vi "Server.vi"() -> ()   [LabVIEW 2023]
uses:
  <vilib>/OPCUA/controls/Data Type.ctl
  <vilib>/OPCUA/controls/NodeId.ctl
  <vilib>/OPCUA/server/Read Variant.vi
  <vilib>/OPCUA/NI OPC UA Server.lvlib
panel:
  out "Temperature on server":variant
  out "Location on server":variant
  in  "Stop Button":bool
  out "Item Node Ids":string
  out "Server Endpoint URL":string
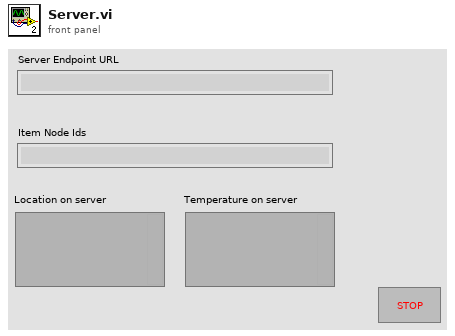
[diagram p1: front panel]
types:
  T1 = typedef "NodeId.ctl" = string
  T2 = typedef "Data Type.ctl" = u16
  T3 = cluster{"name":string, "data type":T2, "access level":u16, "description":string}
  T4 = typedef "OPC UA Server Refnum.ctl" = refnum<k21>
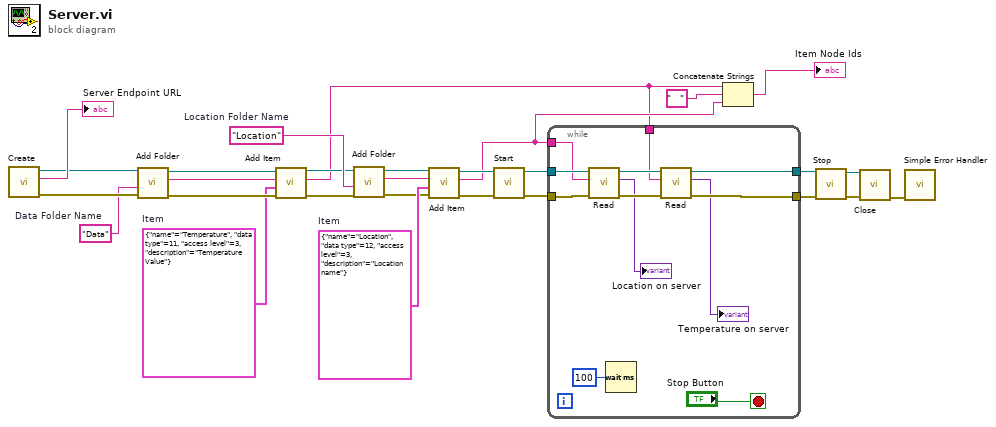
[diagram p0: block diagram]
diagram:
  w8 = "Location"  # Location Folder Name
  w13 = T3 {"name"="Location", "data type"=12, "access level"=3, "description"="Location name"}  # Item
  w16 = T3 {"name"="Temperature", "data type"=11, "access level"=3, "description"="Temperature Value"}  # Item
  w18 = "Data"  # Data Folder Name
  n1 = call <vilib>:"Create.vi"() -> ("error out"=w27:errorcluster, "server endpoint URL"=→"Server Endpoint URL":string, "OPC UA server refnum out"=w21:T4)  [unwired: 9 in]
  n2 = call <vilib>:"Add Folder.vi"("error in (no error)"=w27, "folder name"=w18, "OPC UA server refnum in"=w21) -> ("error out"=w22:errorcluster, "folder node ID"=w17:T1, "OPC UA server refnum out"=w20:T4)  [unwired: 5 in]
  n3 = call <vilib>:"Add Item.vi"("error in (no error)"=w22, "item"=w16, "parent folder node ID"=w17, "OPC UA server refnum in"=w20) -> ("error out"=w10:errorcluster, "item node ID"=w1:T1, "OPC UA server refnum out"=w7:T4)  [unwired: 3 in, 1 out]
  n4 = call <vilib>:"Add Folder.vi"("error in (no error)"=w10, "folder name"=w8, "OPC UA server refnum in"=w7) -> ("error out"=w9:errorcluster, "folder node ID"=w5:T1, "OPC UA server refnum out"=w6:T4)  [unwired: 5 in]
  n5 = call <vilib>:"Add Item.vi"("error in (no error)"=w9, "item"=w13, "parent folder node ID"=w5, "OPC UA server refnum in"=w6) -> ("error out"=w11:errorcluster, "item node ID"=w2:T1, "OPC UA server refnum out"=w12:T4)  [unwired: 3 in, 1 out]
  n6 = call <vilib>:"Start.vi"("error in (no error)"=w11, "OPC UA server refnum in"=w12) -> ("error out"=w15:errorcluster, "OPC UA server refnum out"=w14:T4)  [unwired: 7 in, 1 out]
  n7 = while {
    tunnel: [w33] -> w23
    tunnel: w15 -> [w38]
    tunnel: [w34] -> w19
    tunnel: w14 -> [w37]
    tunnel: w2 -> [w32]
    tunnel: w1 -> [w30]
    stop <- "Stop Button" stop-if-true
    n8 = call-poly <vilib>:"Read.vi"("error in (no error)"=w38, "node ID"=w32, "OPC UA server refnum in"=w37) -> ("error out"=w35:errorcluster, "value"=→"Location on server":variant, "OPC UA server refnum out"=w36:T4)  [unwired: 4 in, 2 out]
    n9 = Wait (ms)(milliseconds to wait=u32 100) -> ()  [unwired: 1 out]
    n10 = call-poly <vilib>:"Read.vi"("error in (no error)"=w35, "node ID"=w30, "OPC UA server refnum in"=w36) -> ("error out"=w33:errorcluster, "value"=→"Temperature on server":variant, "OPC UA server refnum out"=w34:T4)  [unwired: 4 in, 2 out]
  }
  n11 = Concatenate Strings(w1, T1 "   " ("string"), w2) -> (→"Item Node Ids":string)
  n12 = call <vilib>:"Stop.vi"("error in (no error)"=w23, "OPC UA server refnum in"=w19) -> ("error out"=w24:errorcluster, "OPC UA server refnum out"=w26:T4)  [unwired: 8 in]
  n13 = call <vilib>:"Close.vi"("error in (no error)"=w24, "OPC UA server refnum in"=w26) -> ("error out"=w25:errorcluster)  [unwired: 9 in]
  n14 = call <vilib>:"Simple Error Handler.vi"("error in (no error)"=w25) -> ()  [unwired: 4 in, 5 out]
